vi "Pseudo GUID.vi"() -> (5 "GUID String":string)   [LabVIEW 2015]
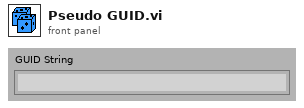
[diagram p1: front panel]
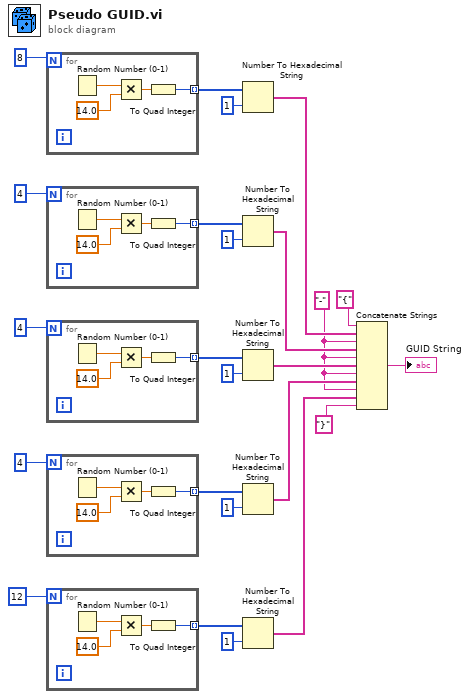
[diagram p0: block diagram]
diagram:
  w2 = "-"
  n1 = for {
    N: 8 -> [_]
    tunnel: [w25] -> w23 mode=indexing
    n2 = Random Number (0-1)() -> (number: 0 to 1=w28:dbl)
    n3 = Multiply(x=w28, y=14.0) -> (x*y=w26:dbl)
    n4 = To Quad Integer(1:w26) -> (0:w25:i64)
  }
  n5 = for {
    N: 4 -> [_]
    tunnel: [w29] -> w20 mode=indexing
    n6 = Random Number (0-1)() -> (number: 0 to 1=w32:dbl)
    n7 = Multiply(x=w32, y=14.0) -> (x*y=w30:dbl)
    n8 = To Quad Integer(1:w30) -> (0:w29:i64)
  }
  n9 = for {
    N: 4 -> [_]
    tunnel: [w33] -> w17 mode=indexing
    n10 = Random Number (0-1)() -> (number: 0 to 1=w36:dbl)
    n11 = Multiply(x=w36, y=14.0) -> (x*y=w34:dbl)
    n12 = To Quad Integer(1:w34) -> (0:w33:i64)
  }
  n13 = for {
    N: 4 -> [_]
    tunnel: [w37] -> w14 mode=indexing
    n14 = Random Number (0-1)() -> (number: 0 to 1=w40:dbl)
    n15 = Multiply(x=w40, y=14.0) -> (x*y=w38:dbl)
    n16 = To Quad Integer(1:w38) -> (0:w37:i64)
  }
  n17 = for {
    N: 12 -> [_]
    tunnel: [w41] -> w11 mode=indexing
    n18 = Random Number (0-1)() -> (number: 0 to 1=w44:dbl)
    n19 = Multiply(x=w44, y=14.0) -> (x*y=w42:dbl)
    n20 = To Quad Integer(1:w42) -> (0:w41:i64)
  }
  n21 = Number To Hexadecimal String(1:i16 1 ("width (-)"), 2:w23) -> (0:w9:string[])
  n22 = Number To Hexadecimal String(1:i16 1 ("width (-)"), 2:w20) -> (0:w8:string[])
  n23 = Number To Hexadecimal String(1:i16 1 ("width (-)"), 2:w17) -> (0:w7:string[])
  n24 = Number To Hexadecimal String(1:i16 1 ("width (-)"), 2:w14) -> (0:w6:string[])
  n25 = Number To Hexadecimal String(1:i16 1 ("width (-)"), 2:w11) -> (0:w5:string[])
  n26 = Concatenate Strings("{", w9, w2, w8, w2, w7, w2, w6, w2, w5, "}") -> (→"GUID String":string)
